vi "Get Battery Stat.vi"(8 "error in (no error)":errorcluster, 10 "nBat":i32, 11 "nSensorIP":u32) -> (0 "error out":errorcluster, 2 "nBat out":i32, 3 "function return":i32)   [LabVIEW 2017, in "imgAcquisiotn.lvlib"]
doc: "DLLFunction int __stdcall ImageCapGetBatteryStat(unsigned int nSensorIP, int* nBat);"
uses:
  imgAcquisiotn.lvlib
  lib/ImageCaptureDLL.dll
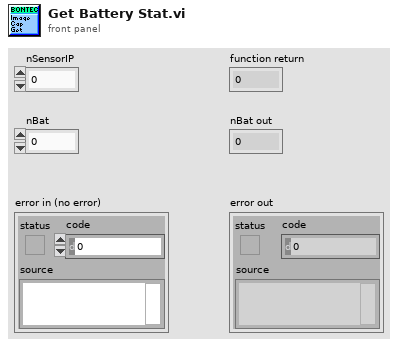
[diagram p1: front panel]
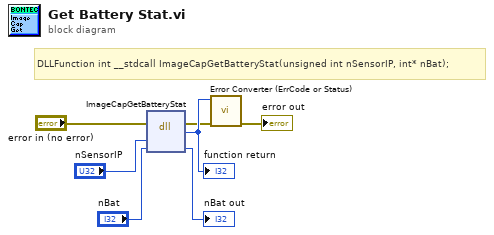
[diagram p0: block diagram]
diagram:
  # "DLLFunction int __stdcall ImageCapGetBatteryStat(unsigned int nSensorIP, int* nBat);"
  n1 = dll-call lib="F:/BonTechFlatPanelLVDriver/lib/ImageCaptureDLL.*" fn="ImageCapGetBatteryStat"(error in="error in (no error)", "nSensorIP"="nSensorIP", "nBat"="nBat") -> (error out=w2:errorcluster, w7:i32, "nBat"=→"nBat out":i32)  [unwired: 3 in, 1 out]
  "function return" <- w7
  n2 = call "Error Converter (ErrCode or Status).vi"("error in (no error)"=w2, "error code"=w7) -> ("error out"=→"error out":errorcluster)  [unwired: 9 in]
